vi "Split TDMS.vi"(8 "error in":errorcluster, 10 "Segments per file":i32, 11 "file path (use dialog)":path) -> (0 "error out":errorcluster)   [LabVIEW 2016]
panel:
  in  "stop":bool
  out "TDMS segment":i32
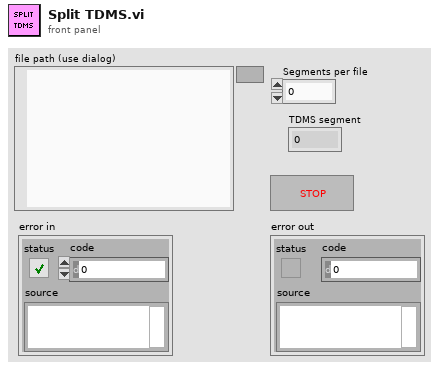
[diagram p1: front panel]
types:
  T1 = enum16{"big-endian, network order", "native, host order", "little-endian"}
  T2 = enum16{"open", "replace", "create", "open or create", "replace or create", "replace or create with confirmation"}
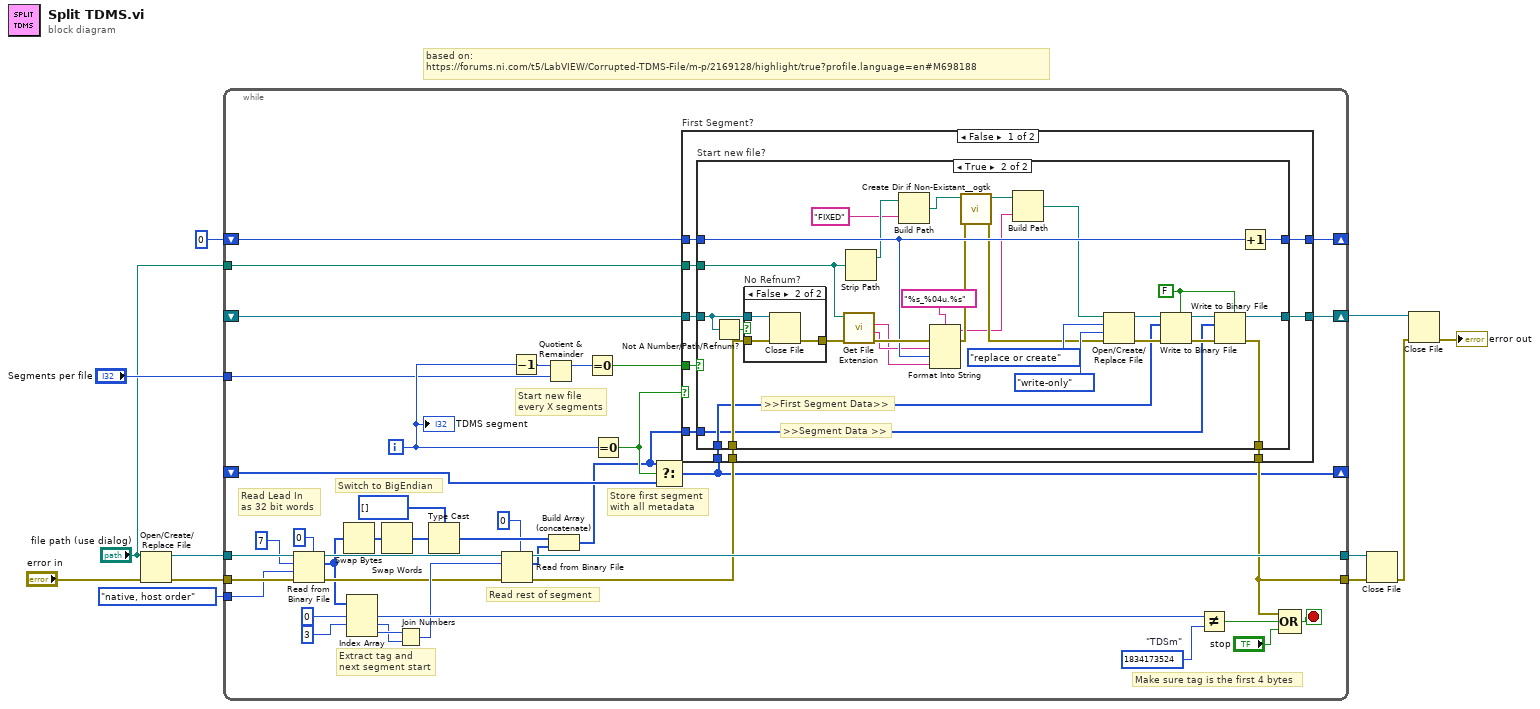
[diagram p0: block diagram]
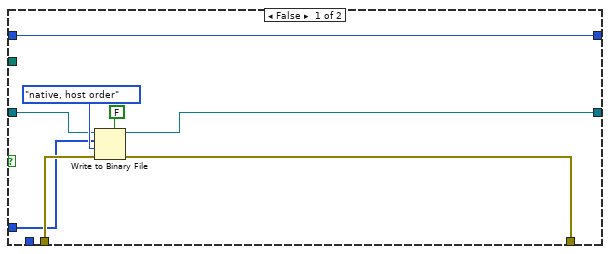
[diagram p2: hidden frame]
diagram:
  # "based on:\nhttps://forums.ni.com/t5/LabVIEW/Corrupted-TDMS-File/m-p/2169128/highlight/true?profile.language=en#M698188"
  n1 = Open/Create/Replace File(file path (use dialog)="file path (use dialog)", error in="error in") -> (refnum out=w11:refnum<file>, error out=w12:errorcluster)  [unwired: 4 in, 1 out]
  n2 = while {
    tunnel: w12 -> [w53]
    tunnel: w11 -> [w52]
    tunnel: T1."native, host order" ("byte order (0:big-endian, network order)") -> [w28]
    tunnel: [w26] -> w9
    tunnel: [w37] -> w8
    shift-right: [w25] -> _
    shift-left: _ -> [w38]
    tunnel: "Segments per file" -> [w31]
    shift-right: [w23] -> w4
    shift-left: _ -> [w22]
    shift-right: [w20] -> _
    shift-left: 0 -> [w21]
    tunnel: "file path (use dialog)" -> [w19]
    i -> [w33]
    stop <- w39 stop-if-true
    w44 = u32 1834173524  # "TDSm"
    # "Switch to BigEndian"
    # "Start new file\nevery X segments"
    # "Store first segment\nwith all metadata"
    # "Make sure tag is the first 4 bytes"
    # "Read rest of segment"
    # "Extract tag and \nnext segment start"
    # "Read Lead In\nas 32 bit words"
    n3 = Read from Binary File(5:u32 0, 8:w53, 9:w28, 10:7 ("count (1)"), 11:w52) -> (0:w40:errorcluster, 2:w15:u32[], 3:w41:refnum<file>)  [unwired: 1 in, 1 out]
    n4 = Swap Bytes(anything=w15) -> (byte swapped=w14:u32[])
    n5 = Index Array(array=w15, index #1=0 ("index"), index #2=3 ("index")) -> (element #1=w45:u32, element #2=w47:u32, element #3=w48:u32)  [unwired: 1 in]
    n6 = Swap Words(1:w14) -> (0:w13:u32[])
    n7 = Join Numbers(hi=w48, lo=w47) -> ((hi.lo)=w42:u64)
    n8 = Type Cast(type=u8[] [], x=w13) -> (*(type *) &x=w35:u8[])
    n9 = Read from Binary File(5:u8 0, 8:w40, 10:w42, 11:w41) -> (0:w27:errorcluster, 2:w36:u8[], 3:w37:refnum<file>)  [unwired: 2 in, 1 out]
    n10 = Decrement(x=w33) -> (x-1=w32:i32)
    n11 = Quotient & Remainder(x=w32, y=w31) -> (x-y*floor(x/y)=w30:i32)  [unwired: 1 out]
    n12 = Build Array (concatenate)(w35, w36) -> (w24:u8[])
    n13 = Equal To 0?(x=w30) -> (x = 0?=w29:bool)
    n14 = Equal To 0?(x=w33) -> (x = 0?=w34:bool)
    n15 = Select(t=w24, s=w34, f=w38) -> (s? t:f=w25:u8[])
    n16 = case "First Segment?" shown="False" w34 {
      tunnel: w29 -> [w63 _]
      tunnel: w27 -> [w62 w108]
      tunnel: [w61 w108] -> w26
      tunnel: w25 -> [w60 _]
      tunnel: w24 -> [w59 _]
      tunnel: [w58 w107] -> w23
      tunnel: w22 -> [w57 w107]
      tunnel: w21 -> [w56 w106]
      tunnel: [w55 w106] -> w20
      tunnel: w19 -> [w54 _]
      frame False {
        n17 = case "Start new file?" shown="True" w63 {
          tunnel: w62 -> [w69 w101]
          tunnel: [w68 w94] -> w61
          tunnel: w60 -> [_ w98]
          tunnel: w59 -> [w67 w92]
          tunnel: [w65 w96] -> w58
          tunnel: w57 -> [w66 w83]
          tunnel: w56 -> [w64 w86]
          tunnel: [w64 w91] -> w55
          tunnel: w54 -> [_ w89]
          frame False {
            n18 = Write to Binary File(file (use dialog)=w66, data=w67, error in=w69, 5:FALSE ("prepend array or string size? (T)"), 9:T1."native, host order" ("byte order (0:big-endian, network order)")) -> (refnum out=w65:refnum<file>, error out=w68:errorcluster)  [unwired: 1 in, 1 out]
          }
          frame True {
            w93 = FALSE ("prepend array or string size? (T)")
            # ">>Segment Data >>"
            # ">>First Segment Data>>"
            n19 = Not A Number/Path/Refnum?(number/path/refnum=w83) -> (NaN/Path/Refnum?=w82:bool)
            n20 = case "No Refnum?" shown="False" w82 {
              tunnel: w83 -> [_ w105]
              tunnel: w101 -> [w102 w104]
              tunnel: [w102 w103] -> w90
              frame True {
              }
              frame False {
                n21 = Close File(refnum=w105, error in=w104) -> (error out=w103:errorcluster)  [unwired: 1 out]
              }
            }
            n22 = call <vilib>:"Get File Extension.vi"("error in (no error)"=w90, "file"=w89) -> ("error out"=w88:errorcluster, "filename without extension"=w85:string, "lowercase file extension"=w84:string)  [unwired: 5 in, 2 out]
            n23 = Strip Path(path=w89) -> (stripped path=w79:path)  [unwired: 1 out]
            n24 = Build Path(base path=w79, name or relative path="FIXED") -> (appended path=w78:path)
            n25 = Format Into String(format string="%s_%04u.%s", error in=w88, w85, w86, w84) -> (resulting string=w72:string, error out=w75:errorcluster)  [unwired: 1 in]
            n26 = call <userlib>:"Create Dir if Non-Existant__ogtk.vi"("error in (no error)"=w75, "Directory Path"=w78) -> ("error out"=w74:errorcluster, "dup Directory Path"=w77:path)  [unwired: 7 in, 1 out]
            n27 = Build Path(base path=w77, name or relative path=w72) -> (appended path=w73:path)
            n28 = Open/Create/Replace File(file path (use dialog)=w73, error in=w74, operation (0:open)=T2."replace or create", access (0:read/write)=enum16{"read/write", "read-only", "write-only"}."write-only") -> (refnum out=w99:refnum<file>, error out=w100:errorcluster)  [unwired: 2 in, 1 out]
            n29 = Write to Binary File(file (use dialog)=w99, data=w98, error in=w100, 5:w93) -> (refnum out=w97:refnum<file>, error out=w95:errorcluster)  [unwired: 2 in, 1 out]
            n30 = Write to Binary File(file (use dialog)=w97, data=w92, error in=w95, 5:w93) -> (refnum out=w96:refnum<file>, error out=w94:errorcluster)  [unwired: 2 in, 1 out]
            n31 = Increment(x=w86) -> (x+1=w91:i32)
          }
        }
      }
      frame True {
        # "Do nothing"
      }
    }
    n32 = Not Equal?(x=w45, y=w44) -> (x != y?=w43:bool)
    n33 = Compound Arithmetic op=OR(w26, w43, "stop") -> (w39:bool)
    "TDMS segment" <- w33
  }
  n34 = Close File(refnum=w8, error in=w9) -> (error out=w3:errorcluster)  [unwired: 1 out]
  n35 = Close File(refnum=w4, error in=w3) -> (error out=→"error out":errorcluster)  [unwired: 1 out]
